vi "Select CSI-2 Data Source.vi"(0 "fpga interface in":refnum<k20>, 5 "csi-2 data source":T1 items=["Raw", "Corrected"], 11 "error in (no error)":errorcluster) -> (4 "fpga interface out":refnum<k20>, 15 "error out":errorcluster)   [LabVIEW 2023, in "GettingStarted_Acq_148X_Host.lvlib"]
uses:
  GettingStarted_Acq_148X_Host.lvlib
  Types/CSI-2 Data Source.ctl
  Types/148x_Acq_FPGA_Reference.ctl
  <vilib>/Utility/error.llb/Error Cluster From Error Code.vi
  <vilib>/rvi/errors/niLvFpgaAdjustHostInterfaceError.vi
  <vilib>/rvi/interface/nirviReadWriteControl/nirviReadWriteControl.xnode
  <vilib>/rvi/interface/Simulation/niFpgaSimulationCallBeginRW.vi
  NiFpgaLv.dll
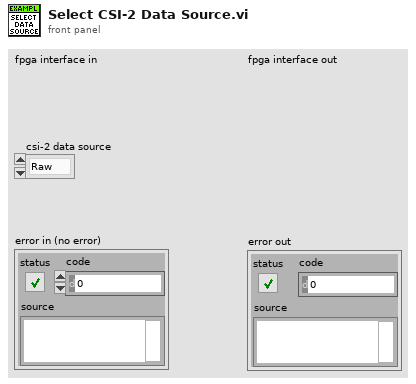
[diagram p1: front panel]
types:
  T1 = typedef "GettingStarted_Acq_148X_Host.lvlib/CSI-2 Data Source.ctl" = u16
  T2 = typedef "GettingStarted_Acq_148X_Host.lvlib/148x_Acq_FPGA_Reference.ctl" = refnum<k20>
  T3 = cluster{"channel acq config":cluster{"stop timeout (cycles)":u32, "first packet data type select mask":u64, "last packet data type select mask":u64, "first and last packet virtual channel must match":bool}, "virtual channel packet filter mask":u16, "data type packet filter mask":u64, "select corrected csi-2 data":bool, "enable channel":bool}[]
  T4 = cluster{"channel acq config":cluster{"stop timeout (cycles)":u32, "first packet data type select mask":u64, "last packet data type select mask":u64, "first and last packet virtual channel must match":bool}, "virtual channel packet filter mask":u16, "data type packet filter mask":u64, "select corrected csi-2 data":bool, "enable channel":bool}
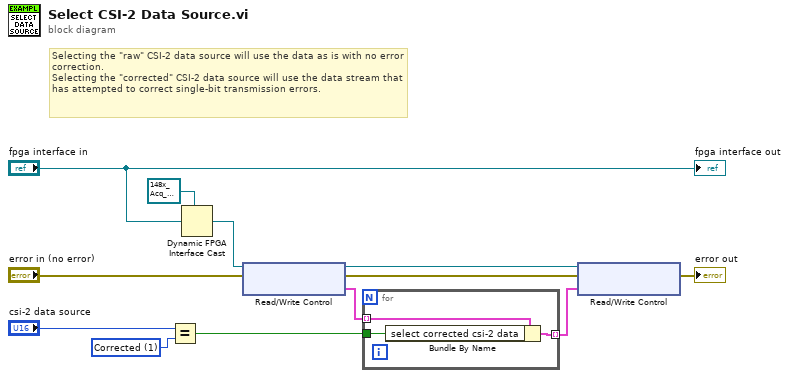
[diagram p0: block diagram]
diagram:
  w9 = T1 1 items=["Raw", "Corrected"] ("csi-2 data source")
  # "Selecting the \"raw\" CSI-2 data source will use the data as is with no error correction.\nSelecting the \"corrected\" CSI-2 data source will use the data stream that has attempted to correct single-bit transmission errors."
  n1 = Equal?(x="csi-2 data source", y=w9) -> (x = y?=w4:bool)
  n2 = Dynamic FPGA Interface Cast(Session In=T2 refnum ("FPGA VI Reference Out"), Type="fpga interface in") -> (Session Out=w2:T2)
  n3 = xnode "Read/Write Control"("FPGA VI Reference In"=w2, "error in"="error in (no error)") -> ("FPGA VI Reference Out"=w6:T2, "error out"=w7:errorcluster, "channel configs"=w8:T3)
  n4 = for {
    tunnel: w8 -> [w15] mode=indexing
    tunnel: w4 -> [w14]
    tunnel: [w13] -> w5 mode=indexing
    n5 = Bundle By Name(cluster=w15, "select corrected csi-2 data"=w14) -> (w13:T4)
  }
  n6 = xnode "Read/Write Control"("FPGA VI Reference In"=w6, "error in"=w7, "channel configs"=w5) -> ("error out"=→"error out":errorcluster)  [unwired: 1 out]
  "fpga interface out" <- "fpga interface in"
